vi "Show.vi"(8 "error in (no error)":errorcluster, 11 "Search Result in":refnum<class "Search Result.lvclass">) -> (0 "error out":errorcluster, 3 "Search Result out":refnum<class "Search Result.lvclass">)   [LabVIEW 2016, in "Better Search.lvlib" / "Search Result.lvclass"]
uses:
  Search Result.lvclass
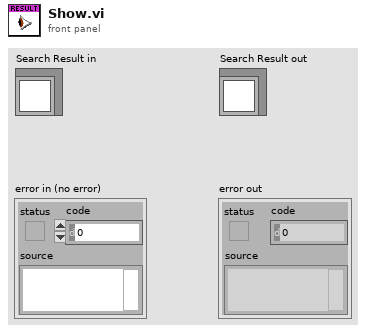
[diagram p1: front panel]
types:
  T1 = enum32{"Invalid", "Standard", "Closed", "Hidden", "Minimized", "Maximized"}
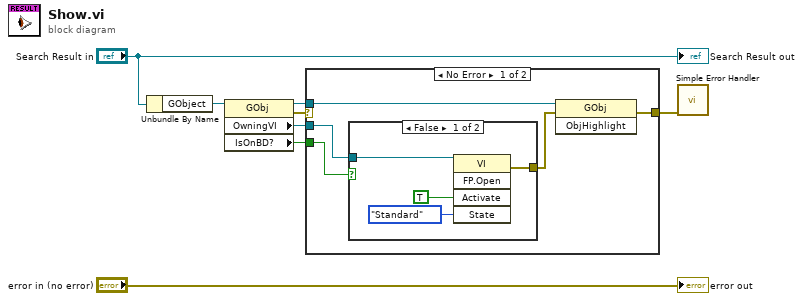
[diagram p0: block diagram]
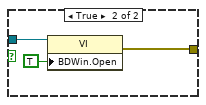
[diagram p2: hidden frame]
diagram:
  n1 = Unbundle By Name("Search Result in") -> ("GObject"=w6:refnum<vi>)
  n2 = property class="GObj"(reference=w6) -> (reference out=w3:refnum<vi>, error out=w1:errorcluster, "OwningVI"=w5:refnum<vi>, "IsOnBD?"=w4:bool)  [unwired: 1 in]
  n3 = case shown="No Error" w1 {
    selector: w1 -> [_ w21]
    tunnel: w5 -> [w13 _]
    tunnel: w4 -> [w12 _]
    tunnel: w3 -> [w11 _]
    tunnel: [w9 w21] -> w2
    frame No Error {
      n4 = case shown="False" w12 {
        tunnel: w13 -> [w17 w20]
        tunnel: [w14 w18] -> w10
        frame False {
          n5 = invoke class="VI" method="FP.Open"(reference=w17, "Activate"=TRUE ("Activate?"), "State"=T1."Standard") -> (error out=w14:errorcluster)  [unwired: 2 in, 4 out]
        }
        frame True {
          n6 = property class="VI"(reference=w20, "BDWin.Open"=TRUE ("Block Diagram Window:Open")) -> (error out=w18:errorcluster)  [unwired: 1 in, 1 out]
        }
      }
      n7 = invoke class="GObj" method="ObjHighlight"(reference=w11, error in=w10) -> (error out=w9:errorcluster)  [unwired: 1 in, 2 out]
    }
    frame Error {
    }
  }
  n8 = call <vilib>:"Simple Error Handler.vi"("error in (no error)"=w2) -> ()  [unwired: 4 in, 5 out]
  "error out" <- "error in (no error)"
  "Search Result out" <- "Search Result in"
